vi "DSF.Engine.Plugin.Tx.Transfer Group.Retrieve Previous.vi"(8 "error in (no error)":errorcluster, 10 "Transfer Group in":refnum<class "DSF.Engine.Transfer Group.lvclass">, 11 "Plugin in":refnum<class "DSF.Engine.Plugin.lvclass">) -> (0 "error out":errorcluster, 2 "Transfer Group out":refnum<class "DSF.Engine.Transfer Group.lvclass">, 3 "Plugin out":refnum<class "DSF.Engine.Plugin.lvclass">)   [LabVIEW 2017, in "DSF.Engine.lvlib" / "DSF.Engine.Plugin.lvclass"]
uses:
  DSF.Engine.Plugin.lvclass
  Transfer/DSF.Engine.Transfer Group.lvclass
  Transfer/DSF.Engine.Transfer Group.lvclass/DSF.Engine.Transfer Group.ctl
  Timing/DSF.Engine.Timing.lvclass/DSF.Engine.Timing.ctl
  Timing/DSF.Engine.Timing.lvclass
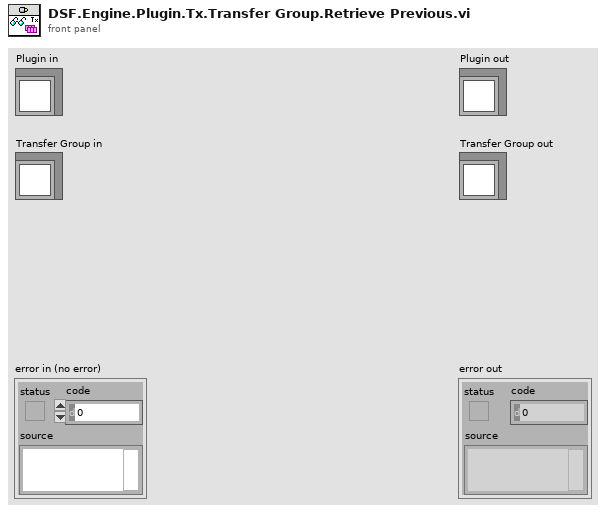
[diagram p1: front panel]
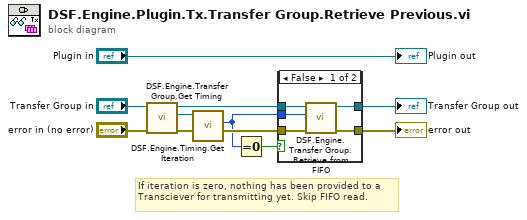
[diagram p0: block diagram]
diagram:
  # "If iteration is zero, nothing has been provided to a Transciever for transmitting yet. Skip FIFO read."
  n1 = call "DSF.Engine.Transfer Group.Get Timing.vi"("Transfer Group in"="Transfer Group in") -> ("Timing"=w3:refnum<class "DSF.Engine.Timing.lvclass">, "Transfer Group out"=w4:refnum<class "DSF.Engine.Transfer Group.lvclass">)  [unwired: 9 in]
  n2 = call "DSF.Engine.Timing.Get Iteration.vi"("Timing in"=w3) -> ("Iteration"=w2:u64)  [unwired: 9 in, 1 out]
  n3 = Equal To 0?(x=w2) -> (x = 0?=w1:bool)
  n4 = case shown="False" w1 {
    tunnel: "error in (no error)" -> [w14 w15]
    tunnel: [w13 w16] -> w8
    tunnel: [w12 w15] -> w7
    tunnel: w4 -> [w11 w16]
    tunnel: w2 -> [w10 _]
    frame False {
      n5 = call "DSF.Engine.Transfer Group.Retrieve from FIFO.vi"("error in (no error)"=w14, "expected iteration"=w10, "Transfer Group in"=w11) -> ("error out"=w12:errorcluster, "Transfer Group out"=w13:refnum<class "DSF.Engine.Transfer Group.lvclass">)  [unwired: 7 in]
    }
    frame True {
    }
  }
  "error out" <- w7
  "Transfer Group out" <- w8
  "Plugin out" <- "Plugin in"
